vi "daqio_Download_File.vi"(8 "error in (no error)":errorcluster, 9 "folder to save the file to":path, 10 "daq.io file ID":string, 11 "daq.io type in":T1={"daq.io ref"=refnum, "daq.io API Base"="http://dashboard.daq.io/api/v1", "Device Type Key"="", "Device Key"="", "Account ID"=""}) -> (0 "error out":errorcluster, 3 "daq.io type out":T1={"daq.io ref"=refnum, "daq.io API Base"="http://dashboard.daq.io/api/v1", "Device Type Key"="", "Device Key"="", "Account ID"=""})   [LabVIEW 2013, in "daqio minimal.lvlib"]
doc: "This VI downloads a specified user file. Please specifiy the file to download by its unique file ID. To retrieve the file IDs you can use the \"Get all Files\" function and search its output array."
uses:
  daqio minimal.lvlib
  _typedefs/daqio-Type.ctl
  <vilib>/httpClient/ClientHandle.ctl
  _typedefs/daqio-File.ctl
  <vilib>/Easy HTTP Client/Easy HTTP.lvlib
  <vilib>/httpClient/LabVIEWHTTPClient.lvlib
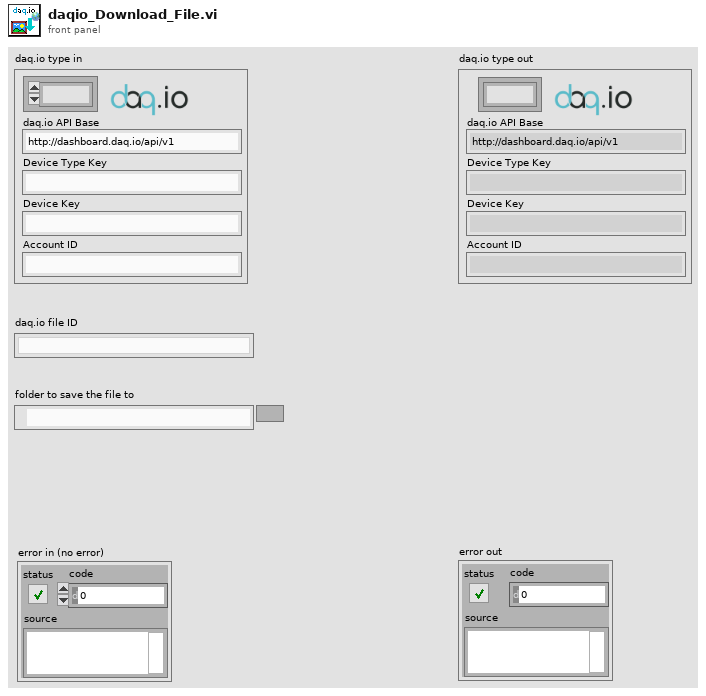
[diagram p1: front panel]
types:
  T1 = typedef "daqio minimal.lvlib/daqio-Type.ctl" = cluster{"daq.io ref":T2, "daq.io API Base":string, "Device Type Key":string, "Device Key":string, "Account ID":string}
  T2 = typedef "LabVIEWHTTPClient.lvlib/ClientHandle.ctl" = refnum<k1>
  T3 = typedef "daqio minimal.lvlib/daqio-File.ctl" = cluster{"id":string, "url":string, "file_type":string, "label":string, "original_file_name":string}
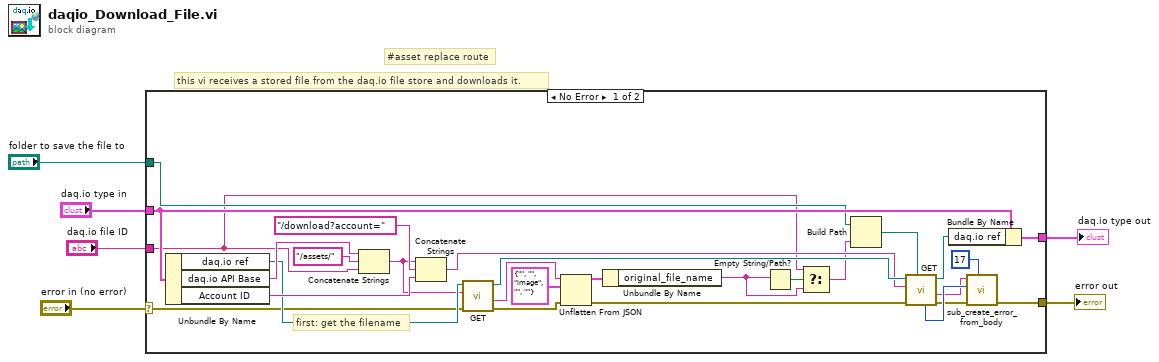
[diagram p0: block diagram]
diagram:
  # "#asset replace route"
  # "this vi receives a stored file from the daq.io file store and downloads it."
  n1 = case shown="No Error" "error in (no error)" {
    selector: "error in (no error)" -> [w26 w35]
    tunnel: "daq.io type in" -> [w31 w36]
    tunnel: [w30 w36] -> w5
    tunnel: [w33 w35] -> w4
    tunnel: "daq.io file ID" -> [w10 _]
    tunnel: "folder to save the file to" -> [w23 _]
    frame No Error {
      # "first: get the filename"
      n2 = Unbundle By Name(w31) -> ("daq.io ref"=w27:T2, "daq.io API Base"=w32:string, "Account ID"=w28:string)
      n3 = Concatenate Strings(w32, "/assets/", w10) -> (w18:string)
      n4 = Concatenate Strings(w18, "/download?account=" ("string"), w28) -> (w19:string)
      n5 = call <vilib>:"GET.vi"("error in (no error)"=w26, "url"=w18, "client handle"=w27) -> ("error out"=w22:errorcluster, "body"=w13:string, "client handle out"=w21:T2)  [unwired: 4 in, 2 out]
      n6 = Unflatten From JSON(JSON string=w13, type and defaults=T3 {"id"="", "url"="", "file_type"="image", "label"="", "original_file_name"=""} ("Asset"), error in (no error)=w22) -> (value=w24:T3, error out=w20:errorcluster)  [unwired: 4 in]
      n7 = Unbundle By Name(w24) -> ("original_file_name"=w11:string)
      n8 = Empty String/Path?(string/path=w11) -> (empty?=w12:bool)
      n9 = Select(t=w10, s=w12, f=w11) -> (s? t:f=w9:string)
      n10 = Build Path(base path=w23, name or relative path=w9) -> (appended path=w15:path)
      n11 = call <vilib>:"GET.vi"("output file"=w15, "error in (no error)"=w20, "url"=w19, "client handle"=w21) -> ("error out"=w14:errorcluster, "body"=w7:string, "client handle out"=w16:T2, "HTTP Response Code"=w17:i32)  [unwired: 3 in, 1 out]
      n12 = Bundle By Name(cluster=w31, "daq.io ref"=w16) -> (w30:T1)
      n13 = call "sub_create_error_from_body.vi"("error code"=17, "error in (no error)"=w14, "http code"=w17, "body"=w7) -> ("error out"=w33:errorcluster)  [unwired: 7 in]
    }
    frame Error {
    }
  }
  "error out" <- w4
  "daq.io type out" <- w5
